vi "Sequence.AddReferences.vi"(8 "error in (no error)":errorcluster, 11 "Sequence":refnum<k24>) -> (0 "error out":errorcluster, 3 "Sequence out":refnum<k24>)   [LabVIEW 2013, in "Simple Sequence Tools - Editor.lvlib"]
uses:
  Simple Sequence Tools - Editor.lvlib
  NationalInstruments.VeriStand.RealTimeSequenceDefinitionApi
  NationalInstruments.VeriStand.Internal
  Shared/SubVIs/Constants.vi
  Shared/Simple Sequence Tools - Shared.lvlib
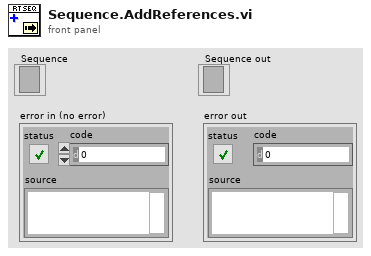
[diagram p1: front panel]
types:
  T1 = typedef "Simple Sequence Tools - Shared.lvlib/Sequence.Reference.ctl" = cluster{"Name":string, "RelativePath":string}
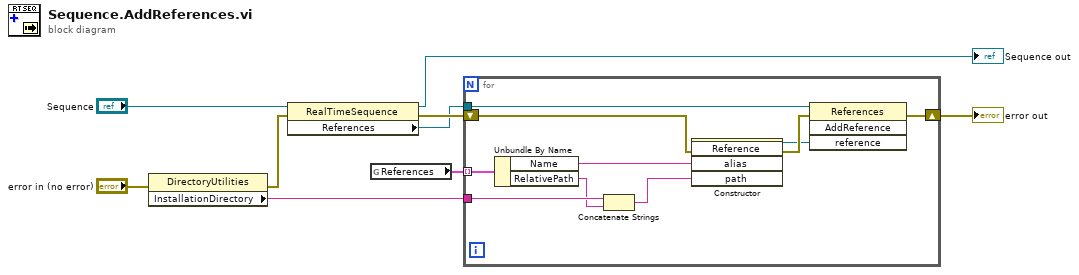
[diagram p0: block diagram]
diagram:
  n1 = property class="DirectoryUtilities"(error in="error in (no error)") -> (error out=w9:errorcluster, "InstallationDirectory"=w7:string)  [unwired: 1 in, 1 out]
  n2 = property class="RealTimeSequence"(reference="Sequence", error in=w9) -> (reference out=→"Sequence out":refnum<k24>, error out=w3:errorcluster, "References"=w2:refnum<k24>)
  n3 = global read "Constants.vi" "References"() -> (w6:T1[])
  n4 = for {
    tunnel: w2 -> [w19]
    shift-right: [w17] -> w5
    shift-left: w3 -> [w16]
    tunnel: w6 -> [w14] mode=indexing
    tunnel: w7 -> [w12]
    n5 = Unbundle By Name(w14) -> ("Name"=w13:string, "RelativePath"=w11:string)
    n6 = Concatenate Strings(w12, w11) -> (w10:string)
    n7 = constructor class="Reference"(error in=w16, "alias"=w13, "path"=w10) -> (reference out=w15:refnum<k24>, error out=w18:errorcluster)  [unwired: 2 in, 3 out]
    n8 = invoke class="References" method="AddReference"(reference=w19, error in=w18, "reference"=w15) -> (error out=w17:errorcluster)  [unwired: 1 in, 3 out]
  }
  "error out" <- w5
